vi "dvp Vi Get Quick Roi Sel Detail.vi"(7 "iSize":i32, 9 "pStrQuickRoi":string, 10 "QuickRoiSel":u32, 11 "handle":u32) -> (1 "pStrQuickRoi out":string, 3 "function return":u32(ring))   [LabVIEW 2018, in "LabViewDVPCamera.lvlib"]
doc: "LabviewDvp2Api dvpStatus dvpViGetQuickRoiSelDetail(\n dvpHandle handle, \n dvpUint32 QuickRoiSel, \n char* pStrQuickRoi,\n int iSize\n );"
uses:
  LabViewDVPCamera.lvlib
  LabViewDVPCamera/LabViewDVPCamera.dll
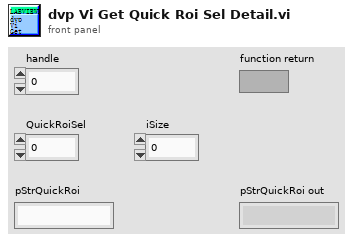
[diagram p1: front panel]
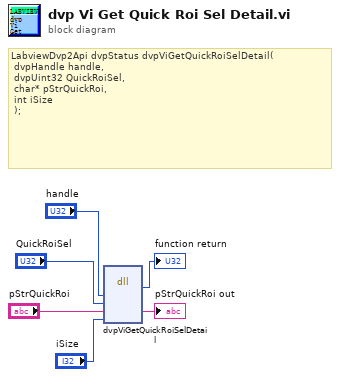
[diagram p0: block diagram]
diagram:
  # "LabviewDvp2Api dvpStatus dvpViGetQuickRoiSelDetail(\n\tdvpHandle handle, \n\tdvpUint32 QuickRoiSel, \n\tchar* pStrQuickRoi,\n\tint iSize\n\t);"
  n1 = dll-call lib="C:/Program Files (x86)/DVP2 Labview cn 64/Sample/LabViewDVPCamera/LabViewDVPCamera.*" fn="dvpViGetQuickRoiSelDetail"("handle"="handle", "QuickRoiSel"="QuickRoiSel", "pStrQuickRoi"="pStrQuickRoi", "iSize"="iSize") -> (→"function return":u32, "pStrQuickRoi"=→"pStrQuickRoi out":string)  [unwired: 6 in, 2 out]
